vi "Set Aout Span.vi"(8 "error in (no error)":errorcluster, 9 "firmware revision":string(combo), 10 "aout span":T2={"ASpanC (20.0)"=20.0, "ASpanL (20.0)"=20.0}, 11 "VISA resource name":refnum<visa-resource-name>) -> (0 "error out":errorcluster, 2 "bridge error":T1, 3 "VISA resource name out":refnum<visa-resource-name>)   [LabVIEW 2020, in "Andeen-Hagerling 2700A.lvlib"]
doc: "Sets the distance between the upper and lower analog output\nvoltage bounds for capacitance and/or loss in volts. These\nanalog output voltage spans correspond directly to the input\ndeviation capacitance and loss spans."
uses:
  Andeen-Hagerling 2700A.lvlib
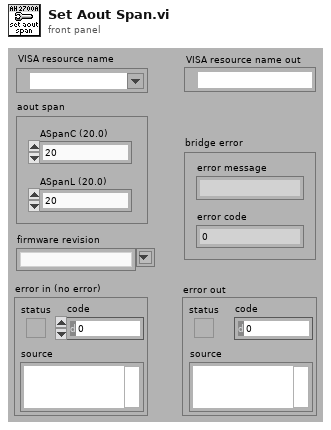
[diagram p1: front panel]
types:
  T1 = cluster{"error message":string, "error code":i32}
  T2 = cluster{"ASpanC (20.0)":dbl, "ASpanL (20.0)":dbl}
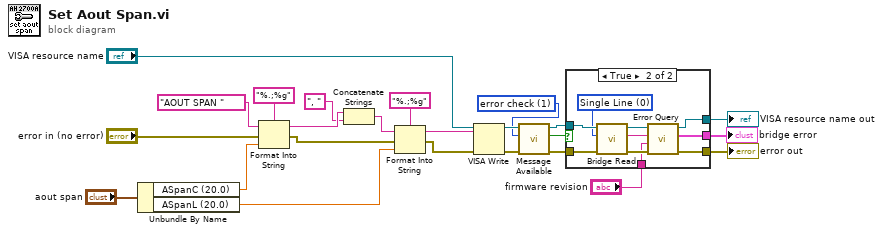
[diagram p0: block diagram]
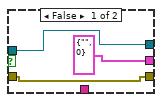
[diagram p2: hidden frame]
diagram:
  w1 = u16 1 items=["none", "error check", "multiline read", "infinite"] ("delay")
  n1 = Unbundle By Name("aout span") -> ("ASpanC (20.0)"=w12:dbl, "ASpanL (20.0)"=w11:dbl)
  n2 = Format Into String(format string="%.;%g", initial string="AOUT SPAN " ("command"), error in="error in (no error)", w12) -> (resulting string=w21:string, error out=w22:errorcluster)
  n3 = Concatenate Strings(w21, ", " ("command")) -> (w15:string)
  n4 = Format Into String(format string="%.;%g", initial string=w15, error in=w22, w11) -> (resulting string=w17:string, error out=w18:errorcluster)
  n5 = VISA Write(VISA resource name="VISA resource name", write buffer=w17, error in (no error)=w18) -> (VISA resource name out=w5:refnum<visa-resource-name>, error out=w4:errorcluster)  [unwired: 1 out]
  n6 = call "Message Available.vi"("error in (no error)"=w4, "delay"=w1, "VISA resource name"=w5) -> ("error out"=w8:errorcluster, "message available"=w10:bool, "VISA resource name out"=w9:refnum<visa-resource-name>)  [unwired: 6 in]
  n7 = case shown="True" w10 {
    tunnel: w9 -> [w26 w34]
    tunnel: w8 -> [w27 w33]
    tunnel: "firmware revision" -> [_ w32]
    tunnel: [w27 w31] -> w2
    tunnel: [w26 w30] -> w3
    tunnel: [T1 {"error message"="", "error code"=0} ("bridge error") w29] -> w6
    frame False {
    }
    frame True {
      w28 = u16 0 items=["Single Line", "Multi-Line"] ("Multiline")
      n8 = call "Bridge Read.vi"("error in (no error)"=w33, "multiline"=w28, "VISA resource name"=w34) -> ("error out"=w36:errorcluster, "read buffer"=w37:string, "VISA resource name out"=w35:refnum<visa-resource-name>)  [unwired: 6 in]
      n9 = call "Error Query.vi"("error in (no error)"=w36, "firmware revision"=w32, "measurement line"=w37, "VISA resource name"=w35) -> ("error out"=w31:errorcluster, "bridge error"=w29:T1, "VISA resource name out"=w30:refnum<visa-resource-name>)  [unwired: 5 in]
    }
  }
  "VISA resource name out" <- w3
  "error out" <- w2
  "bridge error" <- w6
